vi "Error Case Select.vi"(0 "MultiErrors in":refnum<class "MultiErrors.lvclass">) -> (1 "MultiErrors out":refnum<class "MultiErrors.lvclass">, 2 "error out":errorcluster)   [LabVIEW 2020, in "VolatusErrorUtilities.lvlib" / "MultiErrors.lvclass"]
uses:
  MultiErrors.lvclass
  MultiErrors.lvclass/MultiErrors.ctl
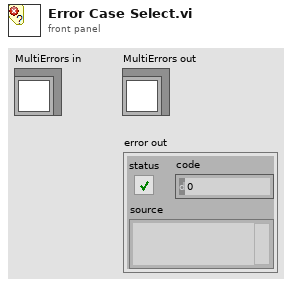
[diagram p1: front panel]
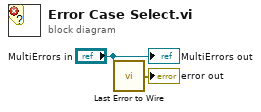
[diagram p0: block diagram]
diagram:
  n1 = call "Last Error to Wire.vi"("MultiErrors in"="MultiErrors in") -> ("error out"=→"error out":errorcluster)  [unwired: 8 in]
  "MultiErrors out" <- "MultiErrors in"
